vi "Add or Edit Wavelengths.vi"(6 "Wavelen in":string[](array[string]), 8 "Ch":i32, 10 "Handle":i32, 11 "OphirLMMeasurementLib.ICoLMMeasurement":refnum<k7>) -> (0 "error out":errorcluster, 2 "Wavelen out":string[](array[string]))   [LabVIEW 2015, in "Powermeter_library.lvlib"]
doc: "Allows the user to add or replace wavelength values for the current channel"
uses:
  Powermeter_library.lvlib
panel:
  in  "Replace":bool
  in  "Add":bool
  in  "New Value:":string
  in  "Wavelengths":i32(listbox)
  # "Outputs"
  # "Inputs"
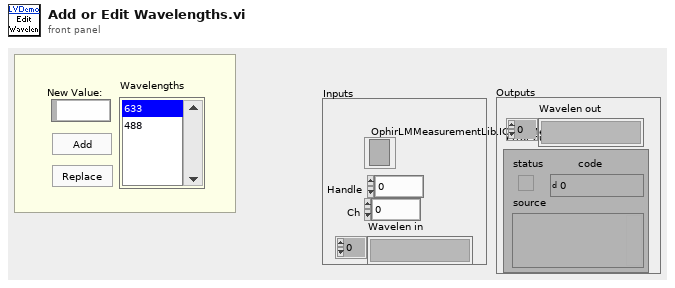
[diagram p1: front panel]
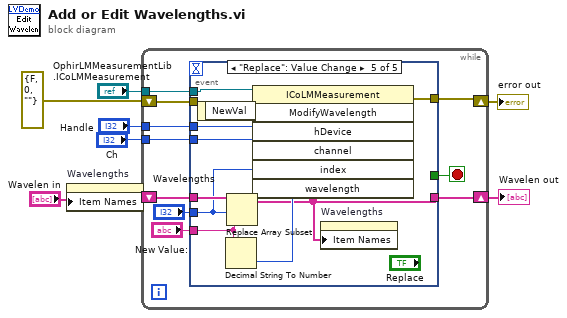
[diagram p0: block diagram]
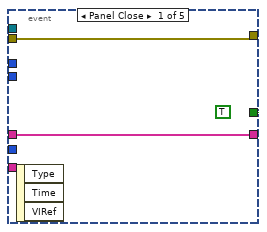
[diagram p2: hidden frame]
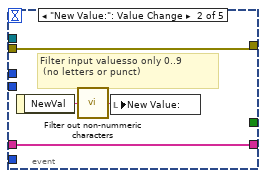
[diagram p3: hidden frame]
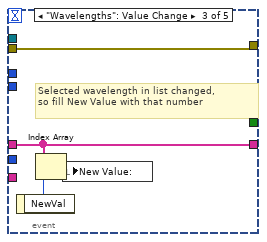
[diagram p4: hidden frame]
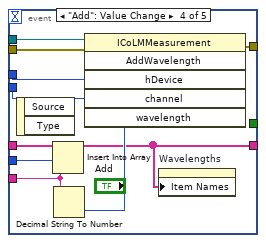
[diagram p5: hidden frame]
diagram:
  n1 = property on="Wavelengths" class="LstBox (strict)"("Item Names"="Wavelen in") -> ()  [unwired: 2 in, 2 out]
  n2 = while {
    shift-right: [w16] -> w6
    shift-left: "Wavelen in" -> [w17]
    tunnel: "OphirLMMeasurementLib.ICoLMMeasurement" -> [w14]
    tunnel: "Handle" -> [w13]
    tunnel: "Ch" -> [w12]
    shift-right: [w9] -> w2
    shift-left: errorcluster {"status"=FALSE, "code"=0, "source"=""} ("error out") -> [w8]
    stop <- w15 stop-if-true
    n3 = event shown="[4] \"Replace\": Value Change" {
      selector: _ -> [_ _ _ _ _]
      dyn-events: _ -> [_ _ _ _ _]
      timeout: _ -> [_ _ _ _ _]
      tunnel: [w20 w24 w28 w31 w39] -> w16
      tunnel: w17 -> [w20 w24 w28 w38 w47]
      tunnel: [TRUE _ _ _ _] -> w15
      tunnel: w14 -> [_ _ _ w36 w46]
      tunnel: w13 -> [_ _ _ w35 w45]
      tunnel: w12 -> [_ _ _ w34 w44]
      tunnel: "Wavelengths" -> [_ _ _ w37 w43]
      tunnel: "New Value:" -> [_ _ _ w33 w42]
      tunnel: [w18 w21 w25 w29 w40] -> w9
      tunnel: w8 -> [w18 w21 w25 w30 _]
      event Panel Close {
        (unwired) TRUE
        n4 = event-data() -> ()  [unwired: 4 out]
      }
      event "New Value:": Value Change {
        # "Filter input valuesso only 0..9\n (no letters or punct)"
        n5 = event-data() -> ("NewVal"=w23:string)  [unwired: 1 out]
        n6 = call "Filter out non-nummeric characters.vi"("string in"=w23) -> ("string out"=w22:string)  [unwired: 6 out]
        n7 = local write "New Value:"(w22) -> ()
      }
      event "Wavelengths": Value Change {
        # "Selected wavelength in list changed,\nso fill New Value with that number"
        n8 = event-data() -> ("NewVal"=w27:i32)  [unwired: 1 out]
        n9 = Index Array(array=w28, index=w27) -> (element=w26:string)
        n10 = local write "New Value:"(w26) -> ()
      }
      event "Add": Value Change {
        n11 = event-data() -> ()  [unwired: 3 out]
        n12 = Insert Into Array(array=w38, index=w37, new element=w33) -> (w31:string[])
        n13 = Decimal String To Number(string=w33) -> (number=w32:i32)  [unwired: 3 out]
        n14 = invoke class="ICoLMMeasurement" method="AddWavelength"(reference=w36, error in=w30, "hDevice"=w35, "channel"=w34, "wavelength"=w32) -> (error out=w29:errorcluster)  [unwired: 1 in, 5 out]
        n15 = property on="Wavelengths" class="LstBox (strict)"("Item Names"=w31) -> ()  [unwired: 2 in, 2 out]
      }
      event "Replace": Value Change {
        n16 = event-data() -> ()  [unwired: 2 out]
        n17 = Decimal String To Number(string=w42) -> (number=w41:i32)  [unwired: 3 out]
        n18 = Replace Array Subset(array=w47, new element=w42, index=w43) -> (w39:string[])
        n19 = invoke class="ICoLMMeasurement" method="ModifyWavelength"(reference=w46, "hDevice"=w45, "channel"=w44, "index"=w43, "wavelength"=w41) -> (error out=w40:errorcluster)  [unwired: 2 in, 6 out]
        n20 = property on="Wavelengths" class="LstBox (strict)"("Item Names"=w39) -> ()  [unwired: 2 in, 2 out]
      }
    }
  }
  "error out" <- w2
  "Wavelen out" <- w6
